vi "VI Tree.vi"   [LabVIEW 2020, in "Keithley 2100 Series.lvlib"]
doc: "This is the instrument driver for the KE2100. The VI Tree displays all the user-callable VIs of the instrument driver in an organized table.\n\nThis VI Tree contains all of the VI's in the LabVIEW template driver. These VI's are intended to be used as starting points for creating your own driver VIs for a particular instrument. Most of these VIs are not operational until they are modified. Rename and save them into your own .LLB file as you modify them for your instrument. ALL National Instrument drivers must include the VI's included in this VI Tree (Initialize, all utility VI's, and Close). You should place all non-user-callable VI's in a utility .LLB. An example of this is the CoreDr_U.LLB file, which contains the non-user-callable VI's for the template driver."
uses:
  Keithley 2100 Series.lvlib
panel:
  # "SEE DIAGRAM\nFOR VI TREE."
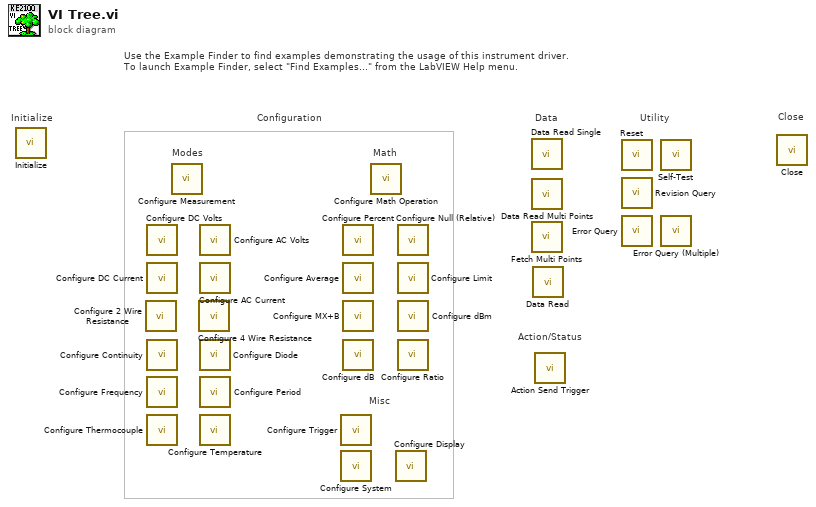
[diagram p0: block diagram]
diagram:
  # "Misc"
  # "Math"
  # "Modes"
  # "Use the Example Finder to find examples demonstrating the usage of this instrument driver.\nTo launch Example Finder, select \"Find Examples...\" from the LabVIEW Help menu."
  # "Configuration"
  # "Utility"
  # "Data"
  # "Action/Status"
  # "Close"
  # "Initialize"
  n1 = call "Initialize.vi"() -> ()  [unwired: 18 in, 2 out]
  n2 = call "Configure 2 Wire Resistance.vi"() -> ()  [unwired: 18 in, 2 out]
  n3 = call "Configure DC Volts.vi"() -> ()  [unwired: 18 in, 2 out]
  n4 = call "Configure DC Current.vi"() -> ()  [unwired: 18 in, 2 out]
  n5 = call "Configure Continuity.vi"() -> ()  [unwired: 18 in, 2 out]
  n6 = call "Configure Frequency.vi"() -> ()  [unwired: 18 in, 2 out]
  n7 = call "Configure Thermocouple.vi"() -> ()  [unwired: 18 in, 2 out]
  n8 = call-poly "Configure Measurement.vi"() -> ()  [unwired: 18 in, 2 out]
  n9 = call "Configure 4 Wire Resistance.vi"() -> ()  [unwired: 18 in, 2 out]
  n10 = call "Configure AC Volts.vi"() -> ()  [unwired: 18 in, 2 out]
  n11 = call "Configure AC Current.vi"() -> ()  [unwired: 18 in, 2 out]
  n12 = call "Configure Diode.vi"() -> ()  [unwired: 18 in, 2 out]
  n13 = call "Configure Period.vi"() -> ()  [unwired: 18 in, 2 out]
  n14 = call "Configure Temperature.vi"() -> ()  [unwired: 18 in, 2 out]
  n15 = call "Configure Trigger.vi"() -> ()  [unwired: 18 in, 2 out]
  n16 = call "Configure System.vi"() -> ()  [unwired: 18 in, 2 out]
  n17 = call "Configure Percent.vi"() -> ()  [unwired: 18 in, 2 out]
  n18 = call "Configure Average.vi"() -> ()  [unwired: 18 in, 2 out]
  n19 = call "Configure MX+B.vi"() -> ()  [unwired: 18 in, 2 out]
  n20 = call "Configure dB.vi"() -> ()  [unwired: 18 in, 2 out]
  n21 = call-poly "Configure Math Operation.vi"() -> ()  [unwired: 18 in, 2 out]
  n22 = call "Configure Display.vi"() -> ()  [unwired: 18 in, 2 out]
  n23 = call "Configure Null (Relative).vi"() -> ()  [unwired: 18 in, 2 out]
  n24 = call "Configure Limit.vi"() -> ()  [unwired: 18 in, 2 out]
  n25 = call "Configure dBm.vi"() -> ()  [unwired: 18 in, 2 out]
  n26 = call "Configure Ratio.vi"() -> ()  [unwired: 18 in, 2 out]
  n27 = call "Data Read Single.vi"() -> ()  [unwired: 17 in, 3 out]
  n28 = call "Data Read Multi Points.vi"() -> ()  [unwired: 17 in, 3 out]
  n29 = call "Fetch Multi Points.vi"() -> ()  [unwired: 17 in, 3 out]
  n30 = call "Data Read.vi"() -> ()  [unwired: 16 in, 4 out]
  n31 = call "Action Send Trigger.vi"() -> ()  [unwired: 18 in, 2 out]
  n32 = call "Reset.vi"() -> ()  [unwired: 18 in, 2 out]
  n33 = call "Revision Query.vi"() -> ()  [unwired: 17 in, 3 out]
  n34 = call "Error Query.vi"() -> ()  [unwired: 16 in, 4 out]
  n35 = call "Self-Test.vi"() -> ()  [unwired: 16 in, 4 out]
  n36 = call "Error Query (Multiple).vi"() -> ()  [unwired: 16 in, 4 out]
  n37 = call "Close.vi"() -> ()  [unwired: 19 in, 1 out]
